vi "teste-global.vi"() -> ()   [LabVIEW 2013]
panel:
  in  "SerialNumber":i32
  out "subarray 2":dbl[](array[numeric])
  out "element":dbl
  out "subarray":dbl[](array[numeric])
  in  "Global Variables":dbl[][](array[numeric])=[[0.0, 0.0], [0.0, 0.0]]
  out "index of element":i32=2
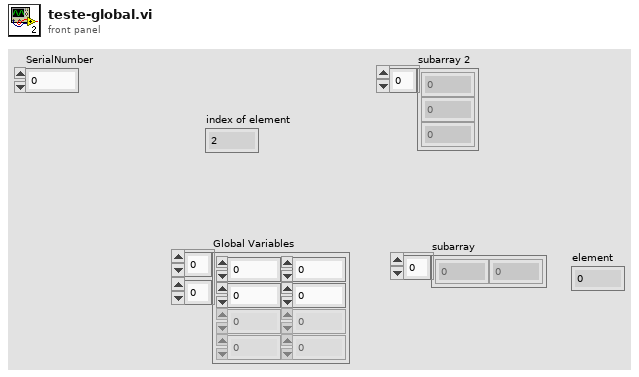
[diagram p1: front panel]
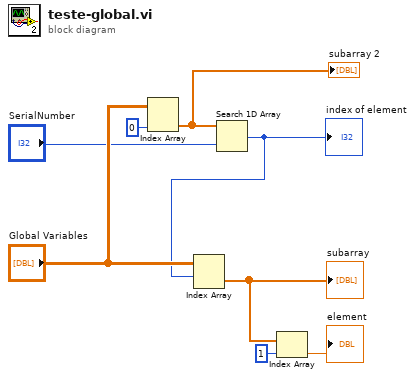
[diagram p0: block diagram]
diagram:
  n1 = Index Array(array="Global Variables", index (col)=0 ("disabled index (col)")) -> (element=w3:dbl[])  [unwired: 1 in]
  "subarray 2" <- w3
  n2 = Search 1D Array(1D array=w3, element="SerialNumber") -> (index of element=w2:i32)  [unwired: 1 in]
  "index of element" <- w2
  n3 = Index Array(array="Global Variables", index (row)=w2) -> (element=w8:dbl[])  [unwired: 1 in]
  "subarray" <- w8
  n4 = Index Array(array=w8, index=1) -> (element=→"element":dbl)
